vi "dfd_Get NStage Rational Filter Param.vi"(6 "fs in":dbl, 7 "factor":T3, 8 "error in (no error)":errorcluster, 9 "ripple specs":T2={"passband"=1.0, "stopband"=60.0, "dB/linear? (T: dB)"=TRUE}, 10 "freq specs":T1={"fpass"=55.0, "fstop"=70.0}, 11 "manual factorization in":T3[](array[typedef])) -> (0 "error out":errorcluster, 1 "ripple specs (dB)":T2={"passband"=0.05437453093312722, "stopband"=0.001, "dB/linear? (T: dB)"=FALSE}, 2 "dup freq specs":T1={"fpass"=55.0, "fstop"=70.0}, 3 "manual factorization out":T3[](array[typedef]), 4 "fs in":dbl, 5 "interpolation/decimation?":bool)   [LabVIEW 2017, in "NI_DigFilterLicensed.lvlib"]
uses:
  <vilib>/addons/Digital Filter Design/NI_DigFilterLicensed.lvlib
  <vilib>/addons/Digital Filter Design/_Objects.llb/DFD Multirate Rational Factor.ctl
  <vilib>/addons/Digital Filter Design/_Objects.llb/DFD Filter Ripple Specification (Design).ctl
  <vilib>/addons/Digital Filter Design/_Objects.llb/DFD Multirate Filter Specification (Design).ctl
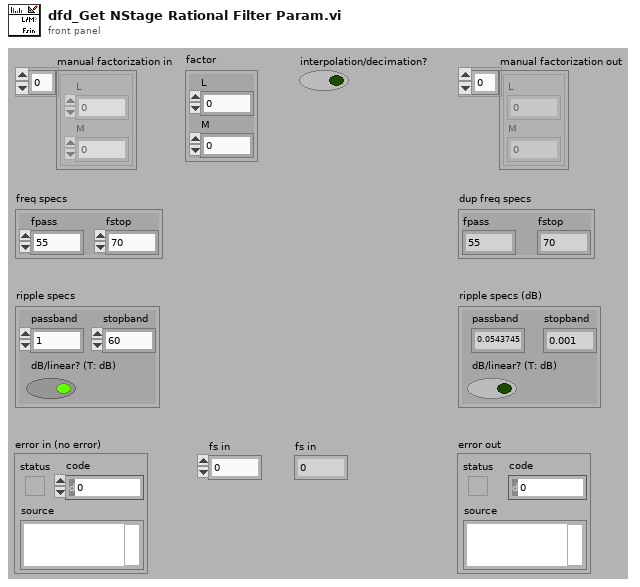
[diagram p1: front panel]
types:
  T1 = typedef "NI_DigFilterLicensed.lvlib/DFD Multirate Filter Specification (Design).ctl" = cluster{"fpass":dbl, "fstop":dbl}
  T2 = typedef "NI_DigFilterLicensed.lvlib/DFD Filter Ripple Specification (Design).ctl" = cluster{"passband":dbl, "stopband":dbl, "dB/linear? (T: dB)":bool}
  T3 = typedef "NI_DigFilterLicensed.lvlib/DFD Multirate Rational Factor.ctl" = cluster{"L":i32, "M":i32}
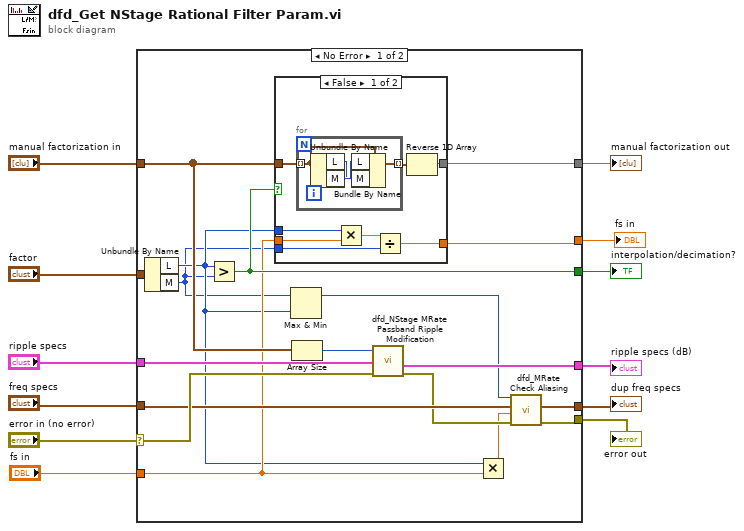
[diagram p0: block diagram]
diagram:
  n1 = case shown="No Error" "error in (no error)" {
    selector: "error in (no error)" -> [w24 w45]
    tunnel: "factor" -> [w30 _]
    tunnel: "fs in" -> [w16 _]
    tunnel: [w17 _] -> w10
    tunnel: [w29 w46] -> w9
    tunnel: [w13 _] -> w8
    tunnel: "manual factorization in" -> [w27 w46]
    tunnel: [w21 w45] -> w2
    tunnel: "ripple specs" -> [w26 _]
    tunnel: [w25 _] -> w5
    tunnel: "freq specs" -> [w23 _]
    tunnel: [w20 _] -> w1
    frame No Error {
      n2 = Unbundle By Name(w30) -> ("L"=w15:i32, "M"=w14:i32)
      n3 = Greater?(x=w15, y=w14) -> (0:w17:bool)
      n4 = case shown="False" w17 {
        tunnel: w27 -> [w38 w44]
        tunnel: [w36 w44] -> w29
        tunnel: w16 -> [w35 w43]
        tunnel: w15 -> [w34 _]
        tunnel: w14 -> [w32 _]
        tunnel: [w31 w43] -> w13
        frame False {
          n5 = for {
            tunnel: w38 -> [w42] mode=indexing
            tunnel: [w39] -> w37 mode=indexing
            n6 = Unbundle By Name(w42) -> ("L"=w40:i32, "M"=w41:i32)
            n7 = Bundle By Name(cluster=w42, "L"=w41, "M"=w40) -> (w39:T3)
          }
          n8 = Multiply(x=w34, y=w35) -> (x*y=w33:dbl)
          n9 = Divide(x=w33, y=w32) -> (x/y=w31:dbl)
          n10 = Reverse 1D Array(array=w37) -> (reversed array=w36:T3[])
        }
        frame True {
        }
      }
      n11 = Max & Min(x=w14, y=w15) -> (max(x,y)=w18:i32)  [unwired: 1 out]
      n12 = Array Size(array=w27) -> (size(s)=w28:i32)
      n13 = call <vilib>:"dfd_NStage MRate Passband Ripple Modification.vi"("error in (no error)"=w24, "ripple specs"=w26, "#stages"=w28) -> ("error out"=w22:errorcluster, "ripple specs (dB)"=w25:T2)  [unwired: 7 out]
      n14 = Multiply(x=w15, y=w16) -> (x*y=w19:dbl)
      n15 = call <vilib>:"dfd_MRate Check Aliasing.vi"("error in"=w22, "fs in [Hz]"=w19, "freq specs"=w23, "factor"=w18) -> ("error out"=w21:errorcluster, "dup freq specs"=w20:T1)  [unwired: 2 in, 4 out]
    }
    frame Error {
    }
  }
  "interpolation/decimation?" <- w10
  "manual factorization out" <- w9
  "fs in" <- w8
  "error out" <- w2
  "ripple specs (dB)" <- w5
  "dup freq specs" <- w1
